vi "EuniceF_Lab7.vi"() -> ()   [LabVIEW 2025]
panel:
  out "Heater":bool
  in  "MODE":bool
  in  "Damping":dbl(slide) scale=0.0..10.0
  in  "SetPoint":dbl(slide) scale=0.0..100.0
  out "Thermistor":dbl(slide) scale=0.0..10.0
  out "HIGH":bool
  out "LOW":bool
  out "Temperature, C":dbl(graph)
  out "Thermometer, C":dbl(slide) scale=0.0..100.0
  in  "stop":bool
  out "AtoD":i16 format="%x"
  out "R,kOhms":dbl(slide) scale=0.0..30.0 scale format="%.2g"
  out "Vscc,V":dbl(slide) scale=0.0..6.0 scale format="%.3g"
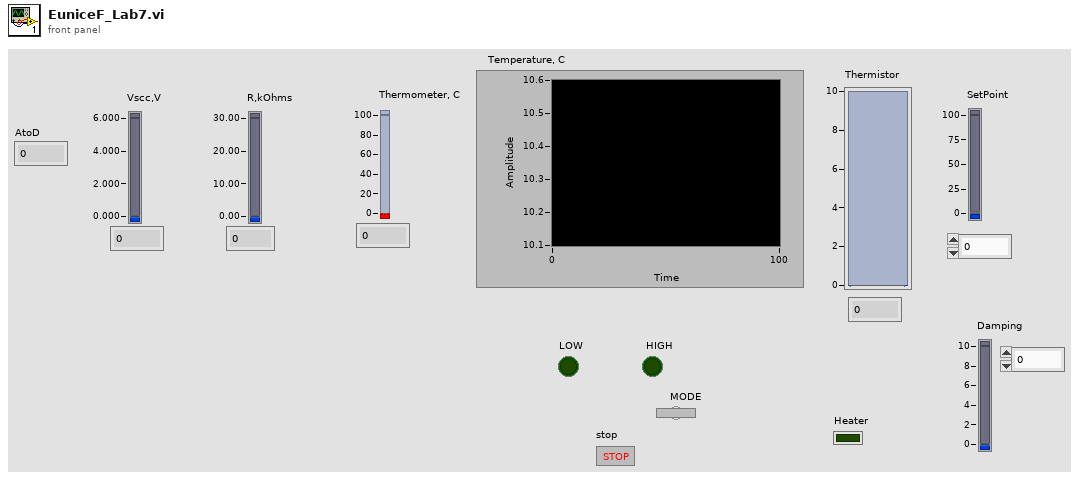
[diagram p1: front panel]
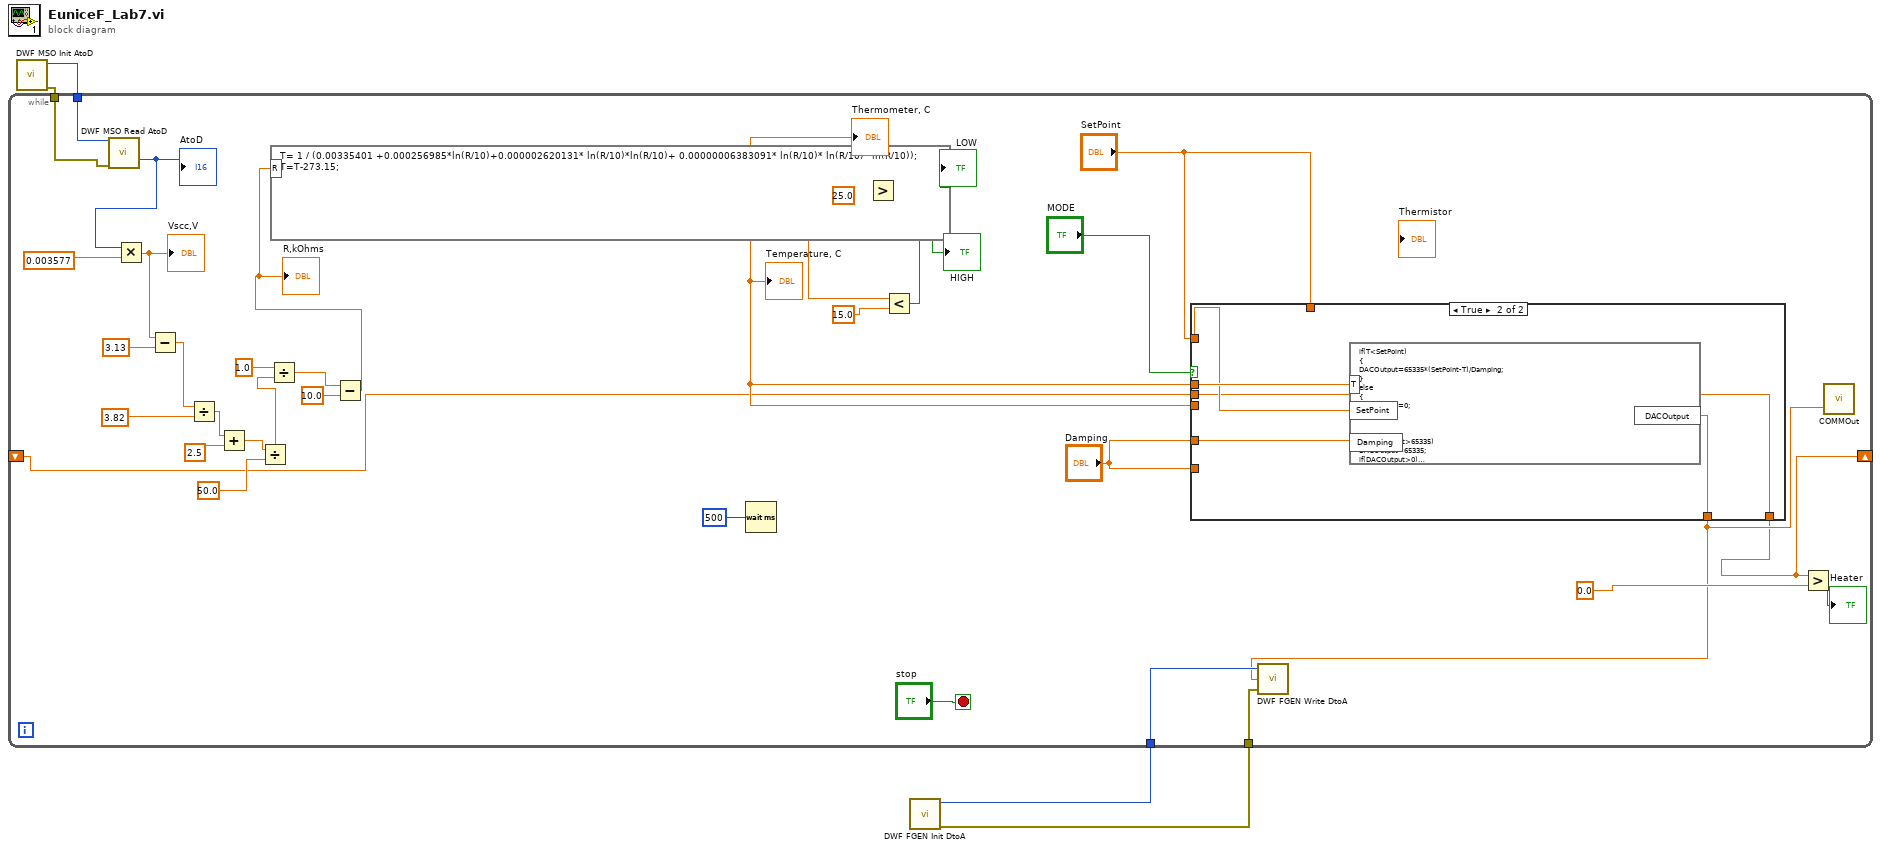
[diagram p0: block diagram]
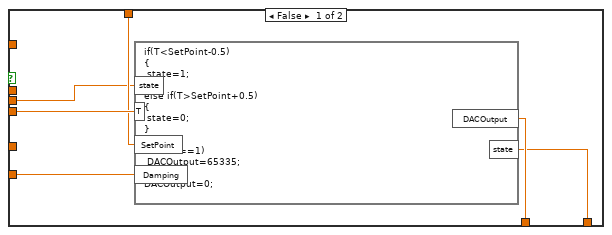
[diagram p2: hidden frame]
diagram:
  n1 = call "DWF MSO Init AtoD.vi"() -> ("Error Out"=w3:errorcluster, "Instrument Handle Out"=w4:i32)  [unwired: 10 in]
  n2 = call "DWF FGEN Init DtoA.vi"() -> ("Error Out"=w1:errorcluster, "Instrument Handle Out"=w2:u32)  [unwired: 10 in]
  n3 = while {
    tunnel: w4 -> [w38]
    tunnel: w3 -> [w37]
    shift-right: [w5] -> _
    shift-left: _ -> [w8]
    tunnel: w2 -> [w15]
    tunnel: w1 -> [w14]
    stop <- "stop" stop-if-true
    n4 = call "DWF MSO Read AtoD.vi"("Instrument Handle In AtoD"=w38, "Error In"=w37) -> ("AtoD"=w36:i16)  [unwired: 12 in, 1 out]
    "AtoD" <- w36
    n5 = Multiply(x=w36, y=0.003577) -> (x*y=w34:dbl)
    "Vscc,V" <- w34
    n6 = Subtract(x=w34, y=3.13) -> (x-y=w31:dbl)
    n7 = Divide(x=w31, y=3.82) -> (x/y=w30:dbl)
    n8 = Add(x=w30, y=2.5) -> (x+y=w28:dbl)
    n9 = Divide(x=w28, y=50.0) -> (x/y=w25:dbl)
    n10 = Divide(x=1.0, y=w25) -> (x/y=w24:dbl)
    n11 = Subtract(x=w24, y=10.0) -> (x-y=w20:dbl)
    "R,kOhms" <- w20
    n12 = formula code="T= 1 / (0.00335401 +0.000256985*ln(R/10)+0.000002620131* ln(R/10)*ln(R/10)+ 0.00000006383091* ln(R/10)* ln(R/10)* ln(R/10));\nT=T-273.15;"("R"=w20) -> ("T"=w11:dbl)
    "Thermometer, C" <- w11
    "Temperature, C" <- w11
    n13 = Wait (ms)(milliseconds to wait=u32 500) -> ()  [unwired: 1 out]
    n14 = Greater?(x=w11, y=25.0) -> (0:→"HIGH":bool)
    n15 = Less?(x=w11, y=15.0) -> (x < y?=→"LOW":bool)
    n16 = case shown="True" "MODE" {
      tunnel: w11 -> [_ w49]
      tunnel: "SetPoint" -> [_ w48]
      tunnel: "Damping" -> [_ w47]
      tunnel: w11 -> [w44 _]
      tunnel: "SetPoint" -> [w43 _]
      tunnel: "Damping" -> [w42 _]
      tunnel: w8 -> [w41 w46]
      tunnel: [w40 w45] -> w7
      tunnel: [w39 w46] -> w5
      frame False {
        n17 = formula code="if(T<SetPoint-0.5)\n{\n state=1;\n}\nelse if(T>SetPoint+0.5)\n{ \n state=0;\n}\n\nif(state==1)\n DACOutput=65335;\nelse\nDACOutput=0;"("T"=w44, "SetPoint"=w43, "Damping"=w42, "state"=w41) -> ("DACOutput"=w40:dbl, "state"=w39:dbl)
      }
      frame True {
        n18 = formula code="if(T<SetPoint)\n{ \nDACOutput=65335*(SetPoint-T)/Damping;\n}\nelse\n{\nDACOutput=0;\n}\n\n\nif(DACOutput>65335)\nDACOutput=65335;\nif(DACOutput>0)\nDACOutput=0;"("T"=w49, "SetPoint"=w48, "Damping"=w47) -> ("DACOutput"=w45:dbl)
      }
    }
    n19 = call "DWF FGEN Write DtoA.vi"("Error In"=w14, "Raw Data"=w7, "Instrument Handle In"=w15) -> ()  [unwired: 1 in, 2 out]
    n20 = Greater?(x=w5, y=0.0) -> (0:→"Heater":bool)
    n21 = call "COMMOut.vi"("Numeric"=w7) -> ()  [unwired: 1 in]
  }
